vi "BundleFlagRoomNumber.vi"(10 "Room Number":i32, 11 "RoomNumFlags":T2={"Flag State"=[1, 3, 5, 7]}) -> (3 "Flags_RoomNum":T1={"Room Number"=0, "RoomNumFlags"={"Flag State"=[1, 3, 5, 7]}})   [LabVIEW 2015]
uses:
  LVClasses/Flags/ColorFlags.ctl
  TypeDef/Flags_RoomNumber.ctl
  LVClasses/Flags/Flags.lvclass
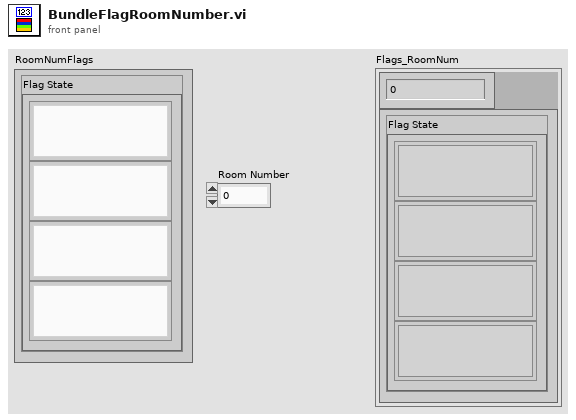
[diagram p1: front panel]
types:
  T1 = typedef "Flags_RoomNumber.ctl" = cluster{"Room Number":i32, "RoomNumFlags":T2}
  T2 = typedef "Flags.lvclass/ColorFlags.ctl" = cluster{"Flag State":u8[]}
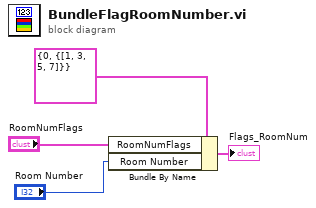
[diagram p0: block diagram]
diagram:
  n1 = Bundle By Name(cluster=T1 {"Room Number"=0, "RoomNumFlags"={"Flag State"=[1, 3, 5, 7]}} ("Flags_RoomNumber"), "RoomNumFlags"="RoomNumFlags", "Room Number"="Room Number") -> (→"Flags_RoomNum":T1)
